vi "Get Selected GU Numbers.vi"(8 "error in":errorcluster, 11 "Listbox Refnum":refnum<vi>) -> (0 "error out":errorcluster, 2 "Selected GU":i32[](array[numeric]))   [LabVIEW 2020, in "GUCalibration2.lvlib"]
uses:
  GUCalibration2.lvlib
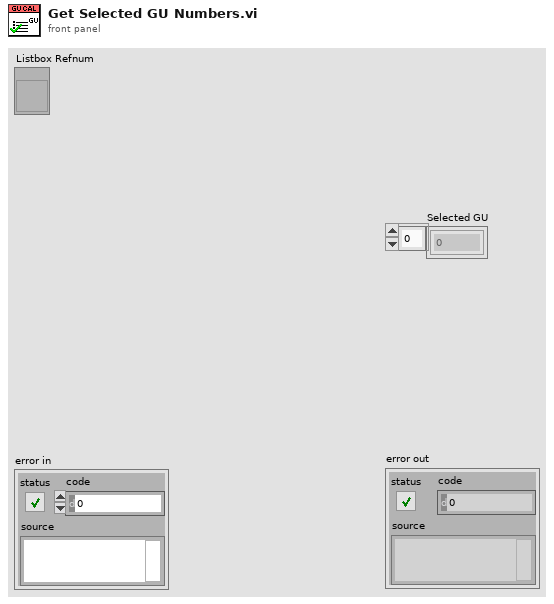
[diagram p1: front panel]
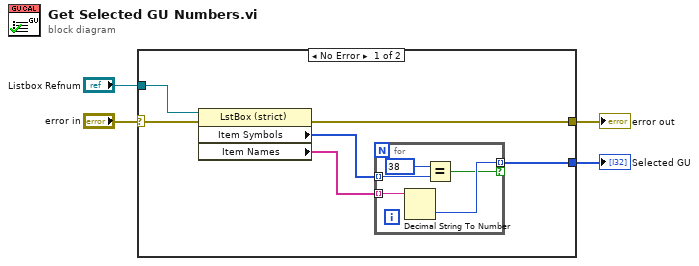
[diagram p0: block diagram]
diagram:
  n1 = case shown="No Error" "error in" {
    selector: "error in" -> [w5 w16]
    tunnel: [w8 w16] -> w4
    tunnel: [w7 _] -> w3
    tunnel: "Listbox Refnum" -> [w6 _]
    frame No Error {
      n2 = property class="LstBox (strict)"(reference=w6, error in=w5) -> (error out=w8:errorcluster, "Item Symbols"=w10:i32[], "Item Names"=w9:string[])  [unwired: 1 out]
      n3 = for {
        tunnel: w9 -> [w13] mode=indexing
        tunnel: w10 -> [w15] mode=indexing
        tunnel: [w12] -> w7 mode=indexing if=w11
        n4 = Decimal String To Number(string=w13) -> (number=w12:i32)  [unwired: 2 in, 1 out]
        n5 = Equal?(x=38, y=w15) -> (x = y?=w11:bool)
      }
    }
    frame Error {
    }
  }
  "error out" <- w4
  "Selected GU" <- w3
